vi "HART_Write command to brooks.vi"(8 "error in":errorcluster, 9 "READ Command":u8, 11 "resource name":refnum<visa-resource-name>) -> (0 "error out":errorcluster)   [LabVIEW 2016]
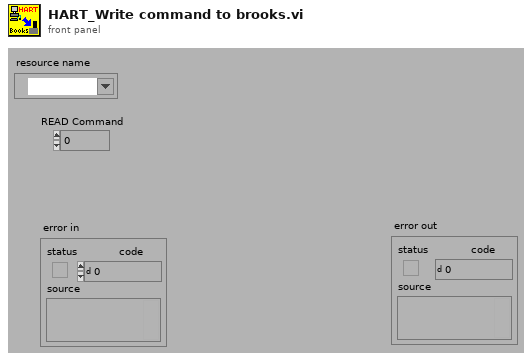
[diagram p1: front panel]
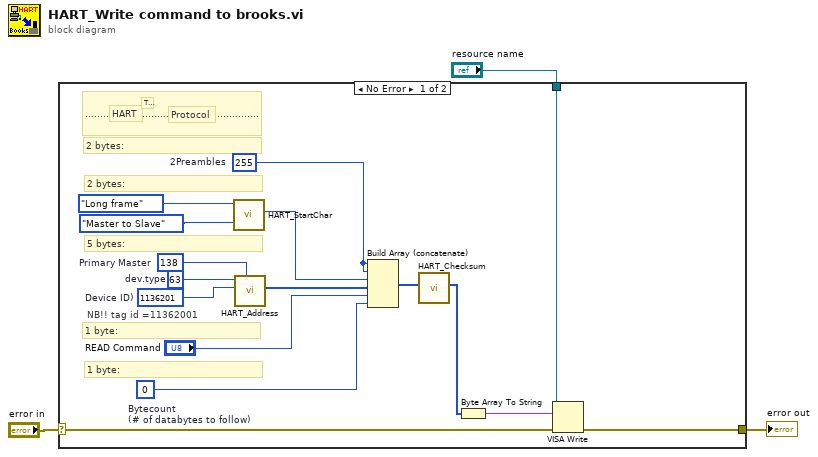
[diagram p0: block diagram]
diagram:
  n1 = case shown="No Error" "error in" {
    selector: "error in" -> [w5 w20]
    tunnel: [w15 w20] -> w3
    tunnel: "resource name" -> [w4 _]
    frame No Error {
      w6 = u8 138  # Primary Master
      w10 = u8 0  # Bytecount (# of databytes to follow)
      w14 = u8 255  # 2Preambles
      w17 = u8 63  # dev.type
      w16 = u32 1136201  # Device ID)
      # "1 byte:"
      # "1 byte:"
      # "5 bytes:"
      # "2 bytes:"
      # "2 bytes:"
      # "Protocol"
      # "TM"
      # "HART"
      # "NB!! tag id =11362001"
      # ".........................................................."
      n2 = call "HART_StartChar.vi"("Message type"=enum16{"Master to Slave", "Slave to Master"}."Master to Slave", "Address type"=enum16{"Short frame", "Long frame"}."Long frame") -> ("start character"=w13:u8)  [unwired: 9 in]
      n3 = call "HART_Address.vi"("Primary Master"=w6, "Tag no. (device ID)"=w16, "Dev Type"=w17) -> ("Address"=w12:u8[])  [unwired: 8 in]
      n4 = Build Array (concatenate)(w14, w14, w13, w12, "READ Command", w10) -> (w9:u8[])
      n5 = call "HART_Checksum.vi"("message"=w9) -> ("message + chk"=w8:u8[])  [unwired: 9 in, 1 out]
      n6 = Byte Array To String(unsigned byte array=w8) -> (string=w7:string)
      n7 = VISA Write(VISA resource name=w4, write buffer=w7, error in (no error)=w5) -> (error out=w15:errorcluster)  [unwired: 2 out]
    }
    frame Error {
    }
  }
  "error out" <- w3
